vi "Read Buffer 0D I32.vi"(8 "error in (no error)":errorcluster, 9 "offset (0)":u64 format="%d bytes", 10 "dst value in":i32, 11 "Buffer in":refnum<class "Buffer.lvclass">) -> (0 "error out":errorcluster, 1 "offset out":u64 format="%d bytes", 2 "dst value out":i32, 3 "Buffer out":refnum<class "Buffer.lvclass">)   [LabVIEW 2017, in "DSF Core.lvlib" / "Buffer.lvclass"]
doc: "Reads from <b>Buffer</b> at the specified <b>offset</b> into <b>dst value</b>."
uses:
  Buffer.lvclass
  C:/Program Files (x86)/National Instruments/LabVIEW 2017/vi.lib/NI/Memory Manager/Classes/Pointer/Pointer.lvclass
  <vilib>/NI/Memory Manager/Classes/Pointer/Pointer.lvclass/Pointer.ctl
  <vilib>/NI/Memory Manager/Classes/Pointer/Read I32.vi
  <vilib>/NI/Memory Manager/Classes/Pointer/Read (No Check).vi
  <vilib>/NI/Memory Manager/Classes/Pointer/Read (No Check) I32.vi
  <vilib>/NI/Memory Manager/Classes/Pointer/Check Move.vi
  <vilib>/NI/Memory Manager/Classes/Pointer/Get Address.vi
  <vilib>/NI/Memory Manager/Classes/Pointer/Check Null Pointer.vi
  <vilib>/NI/Memory Manager/Classes/Pointer/Check Count.vi
  <vilib>/NI/Memory Manager/Classes/Pointer/Check Bounds (Power of 2).vi
  <vilib>/NI/Memory Manager/Classes/Pointer/Errors.vi
  <vilib>/NI/Memory Manager/Classes/Pointer/Null Pointer.vi
  <vilib>/NI/Memory Manager/Classes/Pointer/Is Null.vi
  <vilib>/NI/Memory Manager/Classes/Pointer/Get Size.vi
  <vilib>/NI/Memory Manager/Classes/Pointer/Out of Bounds.vi
  <vilib>/NI/Memory Manager/Classes/Pointer/Check Bounds.vi
  <vilib>/NI/Memory Manager/Classes/Pointer/Create Error.vi
  <vilib>/NI/Memory Manager/Classes/Pointer/Write Pointer Size to Error.vi
  <vilib>/NI/Memory Manager/Classes/Pointer/Check Bounds (Pointer).vi
  <vilib>/NI/Memory Manager/Classes/Pointer/Check Bounds (Buffer).vi
  <vilib>/NI/Memory Manager/Constants/Constants.vi
  <vilib>/NI/Memory Manager/Constants/Library Name.vi
  <vilib>/NI/Memory Manager/Classes/Pointer/Pointer Error Info.vi
  <vilib>/NI/Memory Manager/Constants/Pointer Class Name.vi
  <vilib>/NI/Memory Manager/Classes/Pointer/Buffer Underflow.vi
  <vilib>/NI/Memory Manager/VIs/New Error Cluster.vi
  <vilib>/NI/Memory Manager/VIs/New Error Cluster (512B).vi
  <vilib>/NI/Memory Manager/VIs/Set Error Status.vi
  <vilib>/NI/Memory Manager/VIs/Set Error Code.vi
  <vilib>/NI/Memory Manager/VIs/Set Error Source.vi
  <vilib>/NI/Memory Manager/VIs/Write String to Source.vi
  <vilib>/NI/Memory Manager/VIs/Write Numeric to Source.vi
  <vilib>/NI/Memory Manager/VIs/Write Numeric Scalar to Source (Base10 U64).vi
  <vilib>/NI/Memory Manager/Classes/Pointer/Pointer.lvclass
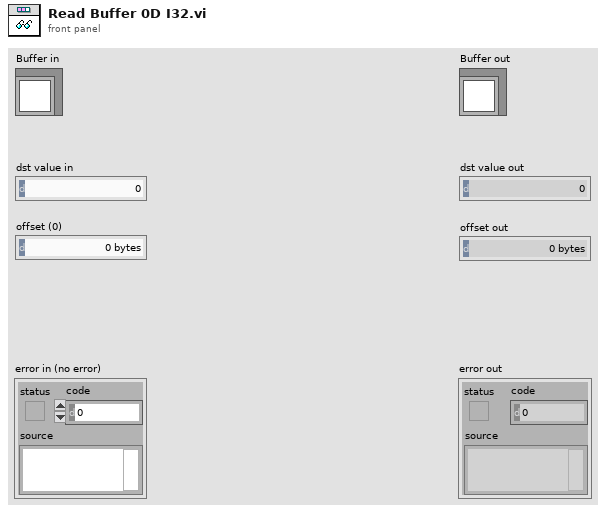
[diagram p1: front panel]
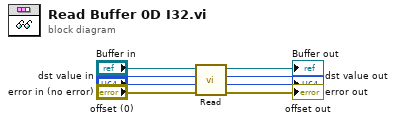
[diagram p0: block diagram]
diagram:
  n1 = call-poly <vilib>:"Read.vi"("error in (no error)"="error in (no error)", "offset (0)"="offset (0)", "value in"="dst value in", "Pointer in"="Buffer in") -> ("error out"=→"error out":errorcluster, "offset out"=→"offset out":u64, "value out"=→"dst value out":i32, "Pointer out"=→"Buffer out":refnum<class "Buffer.lvclass">)  [unwired: 4 in]
